vi "Search 1D Array for Nearest LV2012.vi"(9 "start index (0)":i32, 10 "desired element":dbl, 11 "1D Array":dbl[](array[numeric])) -> (1 "closest index":i32, 3 "closest element":dbl)   [LabVIEW 2012]
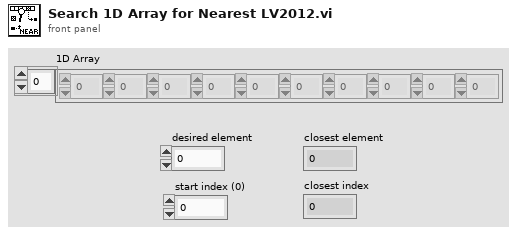
[diagram p1: front panel]
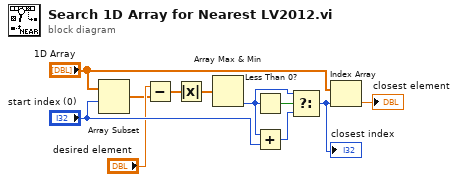
[diagram p0: block diagram]
diagram:
  n1 = Array Subset(array="1D Array", index="start index (0)") -> (w3:dbl[])  [unwired: 1 in]
  n2 = Subtract(x="desired element", y=w3) -> (x-y=w11:dbl[])
  n3 = Absolute Value(x=w11) -> (abs(x)=w8:dbl[])
  n4 = Array Max & Min(array=w8) -> (min index (indices)=w6:i32)  [unwired: 3 out]
  n5 = Less Than 0?(x=w6) -> (x < 0?=w7:bool)
  n6 = Add(x=w6, y="start index (0)") -> (x+y=w5:i32)
  n7 = Select(t=w6, s=w7, f=w5) -> (s? t:f=w1:i32)
  "closest index" <- w1
  n8 = Index Array(array="1D Array", index=w1) -> (element=→"closest element":dbl)
